vi "Set Default Alignment and Line Spacing.vi"(0 "PDF Report IN":refnum<class "PDF Report Class.lvclass">, 1 "Default Paragraph":T1={" Aligment"=enum."JUSTIFY", "Line spacing"=enum."1.0"}, 11 "error in (no error)":errorcluster) -> (4 "PDF Report IN":refnum<class "PDF Report Class.lvclass">, 15 "error out":errorcluster)   [LabVIEW 2019]
doc: "Set the default font of the PDF report.\n\n<B>FRANÇAIS</B>\nChange la police de caractères par défaut du rapport PDF.\n\nVersion 1.0\nDeveloped by Jean-Marc Simard\nCopyright © 2010, Exaprom Inc.\nAll rights reserved.\nLicense: BSD"
uses:
  <userlib>/Exaprom PDF/LV Class/PDF Report Class/PDF Report Class.lvclass
  <userlib>/Exaprom PDF/Controls/Initialization Controls/Defaut Paragraphe and Line Spacing.ctl
  <userlib>/Exaprom PDF/Controls/Text Controls/Texte alignement.ctl
  <userlib>/Exaprom PDF/Controls/Text Controls/Line spacing.ctl
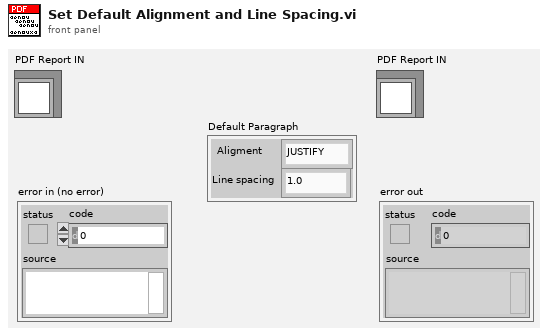
[diagram p1: front panel]
types:
  T1 = typedef "Defaut Paragraphe and Line Spacing.ctl" = cluster{" Aligment":T2, "Line spacing":T3}
  T2 = typedef "Texte alignement.ctl" = enum16{"Select", "CENTER", "JUSTIFY", "LEFT", "RIGHT"}
  T3 = typedef "Line spacing.ctl" = enum16{"Select", "1.0", "1.5", "2.0"}
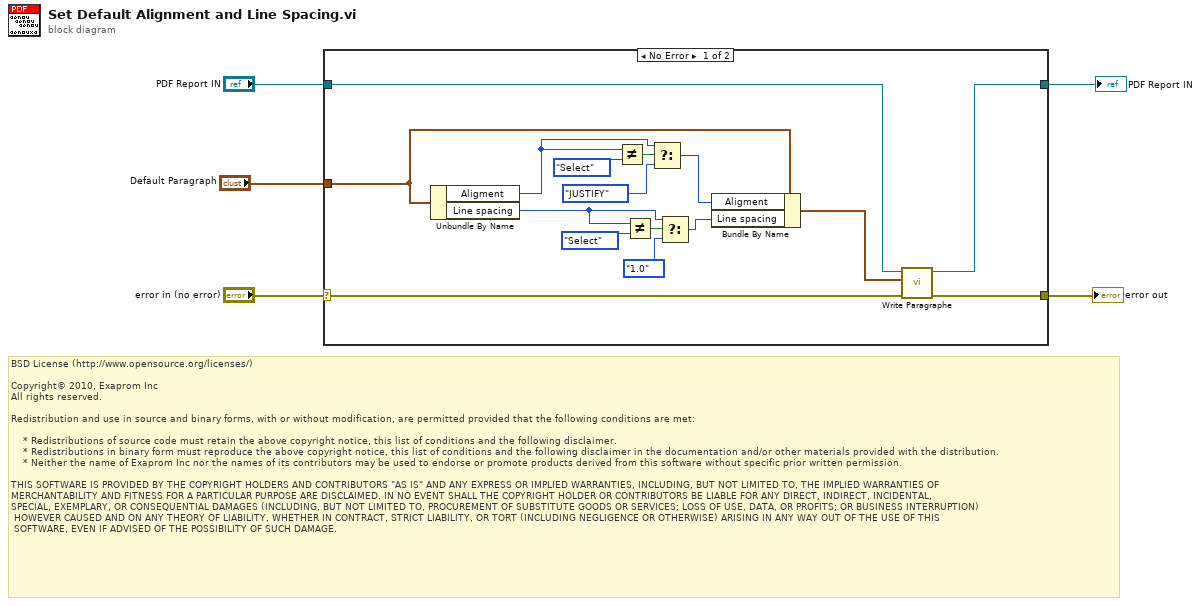
[diagram p0: block diagram]
diagram:
  # "BSD License (http://www.opensource.org/licenses/)\n\nCopyright© 2010, Exaprom Inc\nAll rights reserved.\n\nRedistribution and use in source and binary forms, with or without modification, are permitted provided that the following conditions are met:\n\n    * Redistributions of source code must retain the above copyright notice, this list of conditions and the following disclaimer.\n    * Redistributions in binary form must reproduce the above copyright notice, this list of conditions and the following disclaimer in the documentation and/or other materials provided with the distribution.\n    * Neither the name of Exaprom Inc nor the names of its contributors may be used to endorse or promote products derived from this software without specific prior written permission.\n\nTHIS SOFTWARE IS PROVIDED BY THE COPYRIGHT HOLDERS AND CONTRIBUTORS \"AS IS\" AND ANY EXPRESS OR IMPLIED WARRANTIES, INCLUDING, BUT NOT LIMITED TO, THE IMPLIED WARRANTIES OF \nMERCHANTABILITY AND FITNESS FOR A PARTICULAR PURPOSE ARE DISCLAIMED. IN NO EVENT SHALL THE COPYRIGHT HOLDER OR CONTRIBUTORS BE LIABLE FOR ANY DIRECT, INDIRECT, INCIDENTAL,\nSPECIAL, EXEMPLARY, OR CONSEQUENTIAL DAMAGES (INCLUDING, BUT NOT LIMITED TO, PROCUREMENT OF SUBSTITUTE GOODS OR SERVICES; LOSS OF USE, DATA, OR PROFITS; OR BUSINESS INTERRUPTION)\n HOWEVER CAUSED AND ON ANY THEORY OF LIABILITY, WHETHER IN CONTRACT, STRICT LIABILITY, OR TORT (INCLUDING NEGLIGENCE OR OTHERWISE) ARISING IN ANY WAY OUT OF THE USE OF THIS\n SOFTWARE, EVEN IF ADVISED OF THE POSSIBILITY OF SUCH DAMAGE."
  n1 = case shown="No Error" "error in (no error)" {
    selector: "error in (no error)" -> [w10 w23]
    tunnel: "PDF Report IN" -> [w7 w22]
    tunnel: [w6 w22] -> w4
    tunnel: [w9 w23] -> w3
    tunnel: "Default Paragraph" -> [w13 _]
    frame No Error {
      n2 = Unbundle By Name(w13) -> ("Aligment"=w15:T2, "Line spacing"=w17:T3)
      n3 = Not Equal?(x=w15, y=Texte_alignement."Select" ("Aligment")) -> (x != y?=w14:bool)
      n4 = Not Equal?(x=w17, y=Line_spacing."Select") -> (x != y?=w16:bool)
      n5 = Select(t=w15, s=w14, f=Texte_alignement."JUSTIFY" ("Aligment")) -> (s? t:f=w20:T2)
      n6 = Select(t=w17, s=w16, f=Line_spacing."1.0" ("y")) -> (s? t:f=w19:T3)
      n7 = Bundle By Name(cluster=w13, "Aligment"=w20, "Line spacing"=w19) -> (w8:T1)
      n8 = call-dynamic "Write Paragraphe.vi"("error in (no error)"=w10, "Paragraphe cluster"=w8, "PDF Report Class in"=w7) -> ("error out"=w9:errorcluster, "PDF Report Class out"=w6:refnum<class "PDF Report Class.lvclass">)  [unwired: 7 in]
    }
    frame Error {
    }
  }
  "error out" <- w3
  "PDF Report IN" <- w4
